vi "Pre Launch Init.vi"(11 "Ex Nested in":refnum<class "gController.lvclass">) -> (0 "error out":errorcluster, 3 "Ex Nested out":refnum<class "gController.lvclass">)   [LabVIEW 2017, in "Controller.lvlib" / "gController.lvclass"]
doc: "(<B>Filename</B>: Actor Framework.lvlib:Actor.lvclass:Pre Launch Init.vi)\n\nDefines behavior that occurs after the Launch Nested Actor method is invoked but before the actor's Actor Core method begins running.\n\nBy default, this method does nothing. A descendant class may override it to define behavior."
uses:
  gController.lvclass
  C:/Program Files (x86)/National Instruments/LabVIEW 2017/vi.lib/MSR Consulting, LLC/General Reuse/SuperActor/SuperActor.lvclass
  C:/Program Files (x86)/National Instruments/LabVIEW 2017/vi.lib/ActorFramework/Actor/Actor.lvclass
  Session/Raw FPGA/FPGA Session.lvclass
  C:/Program Files (x86)/National Instruments/LabVIEW 2017/vi.lib/MSR Consulting, LLC/General Reuse/Session APIs/_Session Fwk/Session - Root.lvclass
  Messages/Change Filter MSG/Change Filter Position MSG.lvclass
  C:/Program Files (x86)/National Instruments/LabVIEW 2017/vi.lib/ActorFramework/Message/Message.lvclass
  Messages/Update Vacuum Pump State MSG/Update Vacuum Pump State MSG.lvclass
  Z:/sw_repo/For Builds/Nicholas/Controller/Messages/Generic Boolean MSG/Generic Boolean Message.lvclass
  Messages/Enable Fan MSG/Enable Fan MSG.lvclass
  Messages/Update Fan Voltage MSG/Update Fan Voltage MSG.lvclass
  Messages/Toggle USB MSG/Toggle USB MSG.lvclass
  Messages/Toggle AC Spare MSG/Toggle AC Spare MSG.lvclass
  Messages/Save Data MSG/Save Data MSG.lvclass
  Sequencer/sequenceState.ctl
  Messages/Change Sequence State MSG/Change Sequence State MSG.lvclass
  Messages/Update Heater DC MSG/Update Heater DC MSG.lvclass
  Data/SOAP Data.lvclass
  C:/Program Files (x86)/National Instruments/LabVIEW 2017/vi.lib/MSR Consulting, LLC/General Reuse/Data/Data.lvclass
  Data/Heater Data/Heater Data.lvclass
  <vilib>/MSR Consulting, LLC/General Reuse/Data/Data.lvclass/Data.ctl
  Messages/Generic Boolean MSG/Generic Boolean Message.lvclass/Generic Boolean Message.ctl
  gController.lvclass/gController.ctl
  <vilib>/MSR Consulting, LLC/General Reuse/SuperActor/SuperActor.lvclass/SuperActor.ctl
  <vilib>/ActorFramework/Actor/Actor.lvclass/Actor.ctl
  <vilib>/ActorFramework/Message Enqueuer/Message Enqueuer.lvclass/Message Enqueuer.ctl
  Messages/Change Filter MSG/Change Filter Position MSG.lvclass/Change Filter Position MSG.ctl
  Messages/Update Fan Voltage MSG/Update Fan Voltage MSG.lvclass/Update Fan Voltage MSG.ctl
  Messages/Change Sequence State MSG/Change Sequence State MSG.lvclass/Change Sequence State MSG.ctl
  Messages/Save Data MSG/Save Data MSG.lvclass/Save Data MSG.ctl
  <vilib>/MSR Consulting, LLC/General Reuse/SuperActor/Read CVT Session.vi
  Write DataMap.vi
  Write FPGA Session.vi
  <vilib>/MSR Consulting, LLC/General Reuse/SuperActor/Write ID.vi
  Messages/Change Filter MSG/Write Cell.vi
  Messages/Generic Boolean MSG/Write Bool.vi
  Messages/Update Fan Voltage MSG/Write Voltage.vi
  Messages/Save Data MSG/Write save_.vi
  Write seq_state.vi
  Messages/Change Sequence State MSG/Write sequence state.vi
  <vilib>/MSR Consulting, LLC/General Reuse/Data/Write Data ID.vi
  <vilib>/MSR Consulting, LLC/General Reuse/Data/Write write time.vi
  <vilib>/ActorFramework/Message Enqueuer/Init from Existing Queue.vi
  <vilib>/ActorFramework/Message Priority Queue/Priority Enqueue.vi
  <vilib>/Utility/config.llb/Read Key (Boolean).vi
  <vilib>/Utility/config.llb/Read Key (Double).vi
  <vilib>/Utility/config.llb/Read Key (U32).vi
  <vilib>/MSR Consulting, LLC/General Reuse/SuperActor/Get Config Ref.vi
  <vilib>/MSR Consulting, LLC/General Reuse/SuperActor/xGlobal Data.vi
  Global DO.vi
  <vilib>/ActorFramework/Message Enqueuer/Message Enqueuer.lvclass
  <vilib>/MSR Consulting, LLC/General Reuse/Session APIs/_Session Fwk/Session - Root.lvclass
  <vilib>/MSR Consulting, LLC/General Reuse/SuperActor/SuperActor.lvclass
  <vilib>/Utility/config.llb/NI_LVConfig.lvlib
  <vilib>/ActorFramework/Actor/Actor.lvclass
  Controller.lvlib
  <vilib>/MSR Consulting, LLC/General Reuse/Session APIs/CVT/CVT.lvclass
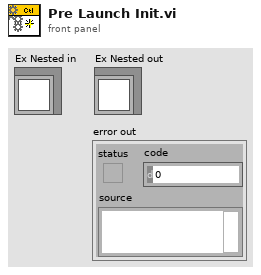
[diagram p1: front panel]
types:
  T1 = typedef "Controller.lvlib/sequenceState.ctl" = enum16{"Run", "Pause", "Reset", "Reload", "Stop"}
  T2 = typedef "Session - Root.lvclass/Session Handle.ctl" = refnum<data-value>
  T3 = typedef "NI_LVConfig.lvlib/Config Data RefNum.ctl" = refnum<k1>
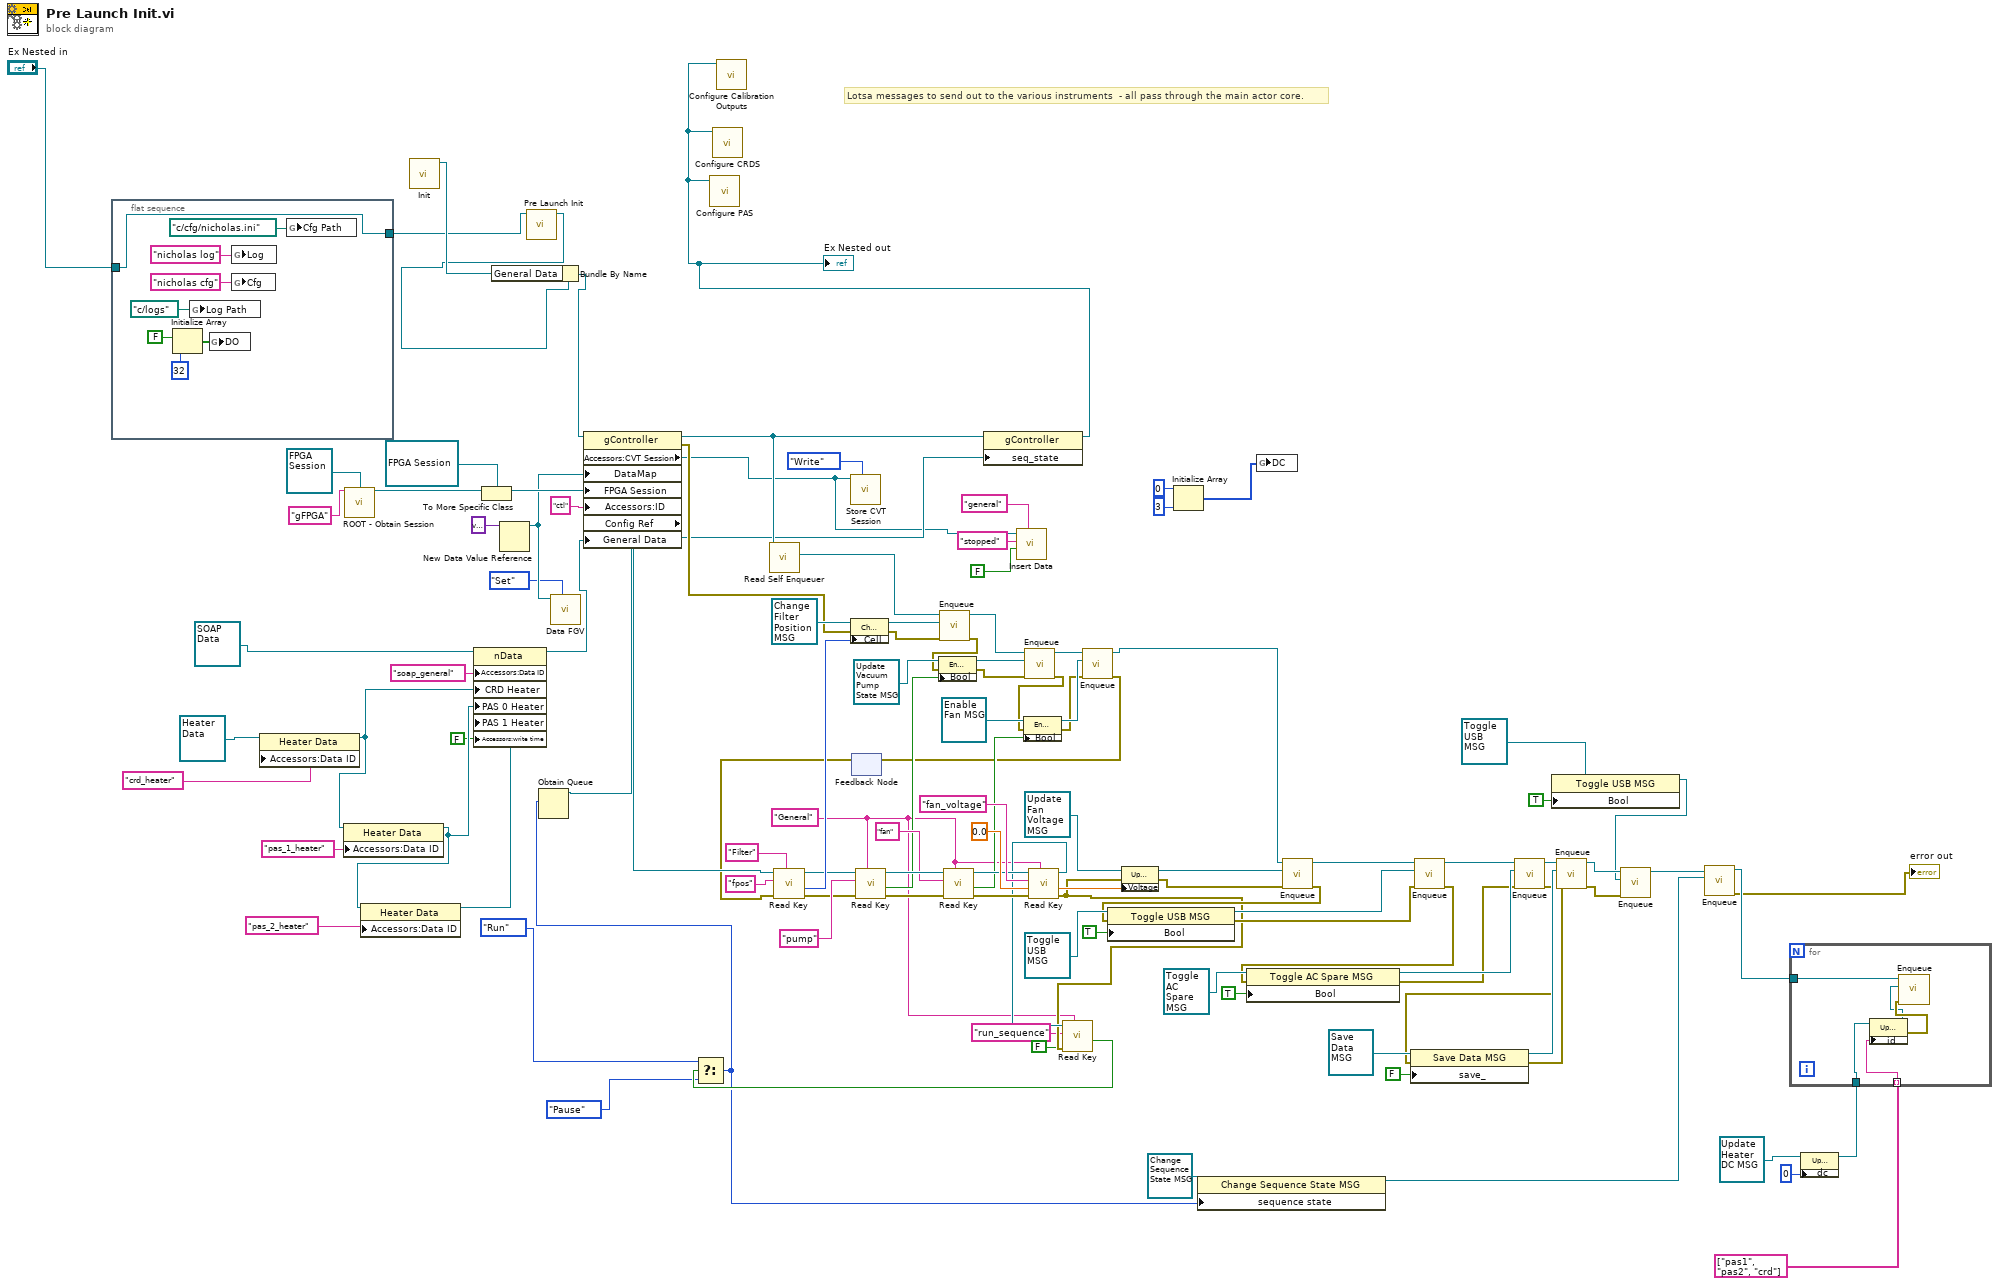
[diagram p0: block diagram]
diagram:
  w42 = "General" ("section")
  # "Lotsa messages to send out to the various instruments  - all pass through the main actor core."
  n1 = flat-sequence {
    tunnel: "Ex Nested in" -> [w119]
    tunnel: [w119] -> w46
    frame #0 {
      n2 = Initialize Array(FALSE, 32 ("dimension size")) -> (w116:bool[])
      n3 = global write "xGlobal Data.vi" "Log Path"(path "c:/logs" ("Cfg Path")) -> ()
      n4 = global write "Global DO.vi" "DO"(w116) -> ()
      n5 = global write "xGlobal Data.vi" "Log"("nicholas log" ("Log")) -> ()
      n6 = global write "xGlobal Data.vi" "Cfg"("nicholas cfg" ("Log")) -> ()
      n7 = global write "xGlobal Data.vi" "Cfg Path"(path "c:/cfg/nicholas.ini" ("Cfg Path")) -> ()
    }
  }
  n8 = property class="Heater Data"(reference=refnum<class "Heater Data.lvclass"> refnum ("Controller.lvlib:Heater Data"), "Accessors:Data ID"="crd_heater" ("Data ID")) -> (reference out=w5:refnum<class "Heater Data.lvclass">)  [unwired: 1 in, 1 out]
  n9 = property class="Heater Data"(reference=w5, "Accessors:Data ID"="pas_1_heater" ("Data ID")) -> (reference out=w4:refnum<class "Heater Data.lvclass">)  [unwired: 1 in, 1 out]
  n10 = call <vilib>:"ROOT - Obtain Session.vi"("Session Name ()"="gFPGA", "OBJ - Session"=refnum<class "FPGA Session.lvclass"> refnum ("FPGA Session")) -> ("Session Handle"=w113:T2)  [unwired: 11 in, 2 out]
  n11 = property class="Heater Data"(reference=w4, "Accessors:Data ID"="pas_2_heater" ("Data ID")) -> (reference out=w3:refnum<class "Heater Data.lvclass">)  [unwired: 1 in, 1 out]
  n12 = call "Init.vi"() -> ("nData out"=w104:refnum<class "SOAP Data.lvclass">)  [unwired: 10 in, 1 out]
  n13 = property class="nData"(reference=refnum<class "SOAP Data.lvclass"> refnum ("Controller.lvlib:nData"), "Accessors:Data ID"="soap_general" ("Data ID"), "CRD Heater"=w5, "PAS 0 Heater"=w4, "PAS 1 Heater"=w3, "Accessors:write time"=FALSE ("write time")) -> (reference out=w2:refnum<class "SOAP Data.lvclass">)  [unwired: 1 in, 1 out]
  n14 = To More Specific Class(target class=refnum<data-value> refnum, reference=w113) -> (specific class reference=w111:refnum<data-value>)  [unwired: 1 in, 1 out]
  n15 = New Data Value Reference(data value=variant) -> (data value reference=w107:refnum<data-value>)  [unwired: 1 in, 1 out]
  n16 = call-parent "Pre Launch Init.vi"("Ex Nested in"=w46) -> ("Ex Nested out"=w45:refnum<class "gController.lvclass">)  [unwired: 9 in, 1 out]
  n17 = Bundle By Name(cluster=w45, "General Data"=w104) -> (w103:refnum<class "gController.lvclass">)
  n18 = call "Data FGV.vi"("Operation"=enum16{"Get", "Set"}."Set", "DataMap"=w107) -> ()  [unwired: 8 in, 2 out]
  n19 = property class="gController"(reference=w103, "DataMap"=w107, "FPGA Session"=w111, "Accessors:ID"="ctl" ("ID"), "General Data"=w2) -> (reference out=w36:refnum<class "gController.lvclass">, error out=w62:errorcluster, "Accessors:CVT Session"=w18:T2, "Config Ref"=w63:T3)  [unwired: 1 in]
  n20 = call <vilib>:"Read Self Enqueuer.vi"("Actor"=w36) -> ("Self Enqueuer"=w64:refnum<class "Message Enqueuer.lvclass">)  [unwired: 10 in]
  n21 = call "Store CVT Session.vi"("Action"=enum16{"Read", "Write"}."Write", "CVT Session In"=w18) -> ()  [unwired: 9 in, 1 out]
  n22 = feedback #1() -> (w55:errorcluster)  [unwired: 1 in]
  n23 = call-poly <vilib>:"Read Key.vi"("section"="Filter", "error in (no error)"=w55, "key"="fpos", "refnum"=w63) -> ("error out"=w54:errorcluster, "value"=w69:u32, "refnum out"=w67:T3)  [unwired: 4 in, 1 out]
  n24 = property class="Change Filter Position"(reference=refnum<class "Change Filter Position MSG.lvclass"> refnum ("Controller.lvlib:Change Filter Position"), error in=w62, "Cell"=w69) -> (reference out=w70:refnum<class "Change Filter Position MSG.lvclass">, error out=w61:errorcluster)
  n25 = call-poly <vilib>:"Read Key.vi"("section"=w42, "error in (no error)"=w54, "key"="pump", "refnum"=w67) -> ("error out"=w77:errorcluster, "value"=w75:bool, "refnum out"=w79:T3)  [unwired: 4 in, 1 out]
  n26 = call <vilib>:"Enqueue.vi"("error in (no error)"=w61, "Message"=w70, "Message Enqueuer in"=w64) -> ("error out"=w60:errorcluster, "Message Enqueuer out"=w73:refnum<class "Message Enqueuer.lvclass">)  [unwired: 7 in]
  n27 = property class="Enable Vacuum Pump MSG"(reference=refnum<class "Update Vacuum Pump State MSG.lvclass"> refnum ("Controller.lvlib:Enable Vacuum Pump MSG"), error in=w60, "Bool"=w75) -> (reference out=w76:refnum<class "Update Vacuum Pump State MSG.lvclass">, error out=w59:errorcluster)
  n28 = call-poly <vilib>:"Read Key.vi"("section"=w42, "error in (no error)"=w77, "key"="fan", "refnum"=w79) -> ("error out"=w85:errorcluster, "value"=w81:bool, "refnum out"=w83:T3)  [unwired: 4 in, 1 out]
  n29 = call <vilib>:"Insert Data.vi"("Group"="general", "Data"=FALSE, "tag"="stopped", "CVT Session In"=w18) -> ()  [unwired: 6 in, 2 out]
  n30 = call <vilib>:"Enqueue.vi"("error in (no error)"=w59, "Message"=w76, "Message Enqueuer in"=w73) -> ("error out"=w58:errorcluster, "Message Enqueuer out"=w102:refnum<class "Message Enqueuer.lvclass">)  [unwired: 7 in]
  n31 = property class="Enable Compressor MSG"(reference=refnum<class "Enable Fan MSG.lvclass"> refnum ("Controller.lvlib:Enable Compressor MSG"), error in=w58, "Bool"=w81) -> (reference out=w82:refnum<class "Enable Fan MSG.lvclass">, error out=w57:errorcluster)
  n32 = call-poly <vilib>:"Read Key.vi"("section"=w42, "error in (no error)"=w85, "default value"=0.0, "key"="fan_voltage", "refnum"=w83) -> ("error out"=w43:errorcluster, "value"=w88:dbl, "refnum out"=w44:T3)  [unwired: 3 in, 1 out]
  n33 = call-poly <vilib>:"Read Key.vi"("section"=w42, "error in (no error)"=w43, "default value"=FALSE, "key"="run_sequence", "refnum"=w44) -> ("value"=w40:bool)  [unwired: 3 in, 3 out]
  n34 = Select(t=sequenceState."Run" ("sequence state"), s=w40, f=sequenceState."Pause" ("sequence state")) -> (s? t:f=w25:T1)
  n35 = Obtain Queue(element data type=w25) -> (queue out=w29:refnum<queue>)  [unwired: 4 in, 2 out]
  n36 = property class="gController"(reference=w36, "seq_state"=w29) -> (reference out=w35:refnum<class "gController.lvclass">)  [unwired: 1 in, 1 out]
  "Ex Nested out" <- w35
  n37 = call "Configure PAS.vi"("Controller In"=w35) -> ()  [unwired: 11 in]
  n38 = call "Configure CRDS.vi"("Controller In"=w35) -> ()  [unwired: 11 in]
  n39 = call "Configure Calibration Outputs.vi"("Controller In"=w35) -> ()  [unwired: 11 in]
  n40 = call <vilib>:"Enqueue.vi"("error in (no error)"=w57, "Message"=w82, "Message Enqueuer in"=w102) -> ("error out"=w56:errorcluster, "Message Enqueuer out"=w65:refnum<class "Message Enqueuer.lvclass">)  [unwired: 7 in]
  n41 = feedback-in #1(w56) -> ()
  n42 = property class="Update Fan Voltage MSG"(reference=refnum<class "Update Fan Voltage MSG.lvclass"> refnum ("Controller.lvlib:Update Fan Voltage MSG"), error in=w43, "Voltage"=w88) -> (reference out=w89:refnum<class "Update Fan Voltage MSG.lvclass">, error out=w53:errorcluster)
  n43 = Initialize Array(u8 0 ("element"), 3 ("dimension size")) -> (w12:u8[])
  n44 = property class="Change Sequence State MSG"(reference=refnum<class "Change Sequence State MSG.lvclass"> refnum ("Controller.lvlib:Change Sequence State MSG"), "sequence state"=w25) -> (reference out=w26:refnum<class "Change Sequence State MSG.lvclass">)  [unwired: 1 in, 1 out]
  n45 = global write "Global DO.vi" "DC"(w12) -> ()
  n46 = call <vilib>:"Enqueue.vi"("error in (no error)"=w53, "Message"=w89, "Message Enqueuer in"=w65) -> ("error out"=w52:errorcluster, "Message Enqueuer out"=w93:refnum<class "Message Enqueuer.lvclass">)  [unwired: 7 in]
  n47 = property class="Toggle USB MSG"(reference=refnum<class "Toggle USB MSG.lvclass"> refnum ("Controller.lvlib:Toggle USB MSG"), error in=w52, "Bool"=TRUE) -> (reference out=w92:refnum<class "Toggle USB MSG.lvclass">, error out=w51:errorcluster)
  n48 = call <vilib>:"Enqueue.vi"("error in (no error)"=w51, "Message"=w92, "Message Enqueuer in"=w93) -> ("error out"=w50:errorcluster, "Message Enqueuer out"=w94:refnum<class "Message Enqueuer.lvclass">)  [unwired: 7 in]
  n49 = property class="Toggle AC Spare MSG"(reference=refnum<class "Toggle AC Spare MSG.lvclass"> refnum ("Controller.lvlib:Toggle AC Spare MSG"), error in=w50, "Bool"=TRUE) -> (reference out=w97:refnum<class "Toggle AC Spare MSG.lvclass">, error out=w49:errorcluster)
  n50 = call <vilib>:"Enqueue.vi"("error in (no error)"=w49, "Message"=w97, "Message Enqueuer in"=w94) -> ("error out"=w48:errorcluster, "Message Enqueuer out"=w98:refnum<class "Message Enqueuer.lvclass">)  [unwired: 7 in]
  n51 = property class="Save Data MSG"(reference=refnum<class "Save Data MSG.lvclass"> refnum ("Controller.lvlib:Save Data MSG"), error in=w48, "save_"=FALSE) -> (reference out=w101:refnum<class "Save Data MSG.lvclass">, error out=w47:errorcluster)
  n52 = property class="Toggle USB MSG"(reference=refnum<class "Toggle USB MSG.lvclass"> refnum ("Controller.lvlib:Toggle USB MSG"), "Bool"=TRUE) -> (reference out=w30:refnum<class "Toggle USB MSG.lvclass">)  [unwired: 1 in, 1 out]
  n53 = call <vilib>:"Enqueue.vi"("error in (no error)"=w47, "Message"=w101, "Message Enqueuer in"=w98) -> ("error out"=w33:errorcluster, "Message Enqueuer out"=w34:refnum<class "Message Enqueuer.lvclass">)  [unwired: 7 in]
  n54 = call <vilib>:"Enqueue.vi"("error in (no error)"=w33, "Message"=w30, "Message Enqueuer in"=w34) -> ("Message Enqueuer out"=w27:refnum<class "Message Enqueuer.lvclass">)  [unwired: 7 in, 1 out]
  n55 = call <vilib>:"Enqueue.vi"("Message"=w26, "Message Enqueuer in"=w27) -> ("error out"=→"error out":errorcluster, "Message Enqueuer out"=w24:refnum<class "Message Enqueuer.lvclass">)  [unwired: 8 in]
  n56 = property class="Update Heater DC MSG"(reference=refnum<class "Update Heater DC MSG.lvclass"> refnum ("Controller.lvlib:Update Heater DC MSG.lvclass"), "dc"=u8 0) -> (reference out=w21:refnum<class "Update Heater DC MSG.lvclass">)  [unwired: 1 in, 1 out]
  n57 = for {
    tunnel: w24 -> [w128]
    tunnel: w21 -> [w126]
    tunnel: string[] ["pas1", "pas2", "crd"] -> [w125] mode=indexing
    n58 = property class="Update Heater DC MSG"(reference=w126, "id"=w125) -> (reference out=w124:refnum<class "Update Heater DC MSG.lvclass">, error out=w127:errorcluster)  [unwired: 1 in]
    n59 = call <vilib>:"Enqueue.vi"("error in (no error)"=w127, "Message"=w124, "Message Enqueuer in"=w128) -> ()  [unwired: 7 in, 2 out]
  }
